vi "TargetCorner_GetAll.vi"(11 "TargetCorner":T1) -> (1 "Y":dbl, 3 "X":dbl)   [LabVIEW 2019, in "PhotonVisionLib.lvlib"]
doc: "Get the individual components of a TargetCorner\n\nInputs:\n - TargetCorner -- TargetCorner cluster\n\nOutputs:\n - X -- \n - Y --"
uses:
  PhotonVisionLib.lvlib
  TypeDef/TargetCornerType.ctl
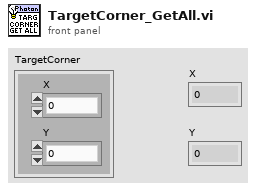
[diagram p1: front panel]
types:
  T1 = typedef "PhotonVisionLib.lvlib/TargetCornerType.ctl" = cluster{"X":dbl, "Y":dbl}
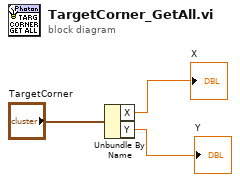
[diagram p0: block diagram]
diagram:
  n1 = Unbundle By Name("TargetCorner") -> ("X"=→"X":dbl, "Y"=→"Y":dbl)
